vi "xxxx.vi"(8 "error in (no error)":errorcluster, 11 "Context in":refnum<class "Context.lvclass">) -> (0 "error out":errorcluster, 3 "Context out":refnum<class "Context.lvclass">)   [LabVIEW 2021, in "Context.lvlib" / "Context.lvclass"]
uses:
  Context.lvclass
  C:/PPLs/Design-Patterns/State Pattern/State Pattern/State Pattern/State Pattern.lvclass
  State/State.lvclass
  State Pattern/State Pattern/State Pattern.lvclass
  Context.lvclass/Context.ctl
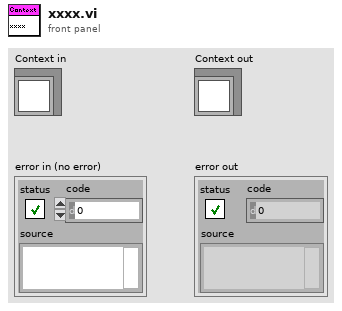
[diagram p1: front panel]
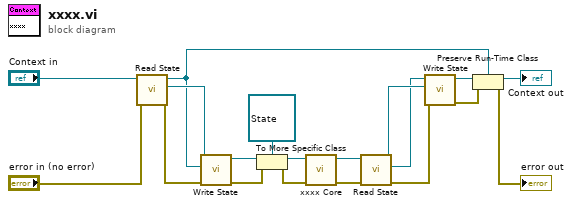
[diagram p0: block diagram]
diagram:
  n1 = call-dynamic "Read State.vi"("error in (no error)"="error in (no error)", "Context in"="Context in") -> ("error out"=w19:errorcluster, "State"=w15:refnum<class "State Pattern.lvclass">, "Context out"=w1:refnum<class "Context.lvclass">)  [unwired: 7 in]
  n2 = call-dynamic "Write State.vi"("error in (no error)"=w19, "State"=w1, "State Pattern in"=w15) -> ("error out"=w11:errorcluster, "State Pattern out"=w14:refnum<class "State Pattern.lvclass">)  [unwired: 7 in]
  n3 = To More Specific Class(target class=refnum<class "State.lvclass"> refnum ("Context.lvlib:Context State.lvclass"), reference=w14, error in=w11) -> (specific class reference=w13:refnum<class "State.lvclass">, error out=w10:errorcluster)
  n4 = call-dynamic "xxxx Core.vi"("error in (no error)"=w10, "State in"=w13) -> ("error out"=w16:errorcluster, "State out"=w17:refnum<class "State.lvclass">)  [unwired: 8 in]
  n5 = call-dynamic "Read State.vi"("error in (no error)"=w16, "State Pattern in"=w17) -> ("error out"=w5:errorcluster, "State"=w3:refnum<class "State Pattern.lvclass">, "State Pattern out"=w18:refnum<class "State.lvclass">)  [unwired: 7 in]
  n6 = call-dynamic "Write State.vi"("error in (no error)"=w5, "State"=w18, "State Pattern in"=w3) -> ("error out"=w8:errorcluster, "State Pattern out"=w2:refnum<class "State Pattern.lvclass">)  [unwired: 7 in]
  n7 = Preserve Run-Time Class(object in=w2, error in=w8, 2:w1) -> (object out=→"Context out":refnum<class "Context.lvclass">, error out=→"error out":errorcluster)
